vi "Trigger Each Line From Encoder (Camera Link).vi"() -> ()   [LabVIEW 2023]
doc: "The Trigger Each Line From Encoder (Camera Link) VI uses the Phase A & B pins from an encoder to trigger the acquisition of each image line. Because the encoder frequency is generally higher than the desired line rate, use the Divide Factor to adjust the Scaled Encoder signal frequency to match that of the desired line rate. The encoder hardware on NI frame grabbers is designed to accomodate backlash, so the Scaled Encoder signal will only pulse for cumulative forward movement of the encoder itself.\n\nNOTE: This example requires a linescan camera with an IMAQdx-supported Camera Link frame grabber. If supported, the Use IO Board Input control determines whether the encoder input lines are sourced from the IO Extension Board or from the front panel IO connector."
uses:
  <vilib>/vision/driver/NI_Vision_Acquisition_Software.lvlib
  <resource>/objmgr/imaqdx.rc
panel:
  in  "Encoder Parameters":T1={"Divide Factor"=10, "Phase A Polarity"=0, "Phase B Polarity"=0, "Phase A & B Filter"=FALSE, "Use IO Board Input"=FALSE} {"Phase B Polarity" items=["Active High", "Active Low"]; "Phase A Polarity" items=["Active High", "Active Low"]}
  in  "Camera Name":refnum<k21> caption="IMAQdx Session"
  out "Buffer Number":u32
  out "Image":T2(plugin-control)
  out "Frame Rate":dbl
  in  "Stop":bool
  # "Overview: Demonstrates how to acquire images continuously using a grab acquisition while triggering each line of an image from an encoder.\nRequirements: Vision Acquisition Software; Camera Link frame grabber; Camera Link line scan camera configured to trigger each line from Camera Control line 1 (CC1); encoder wired to the encoder input of the frame grabber\nInstructions: \n1. Select the Camera Name.\n2. Configure the encoder parameters.\n3. Run the VI"
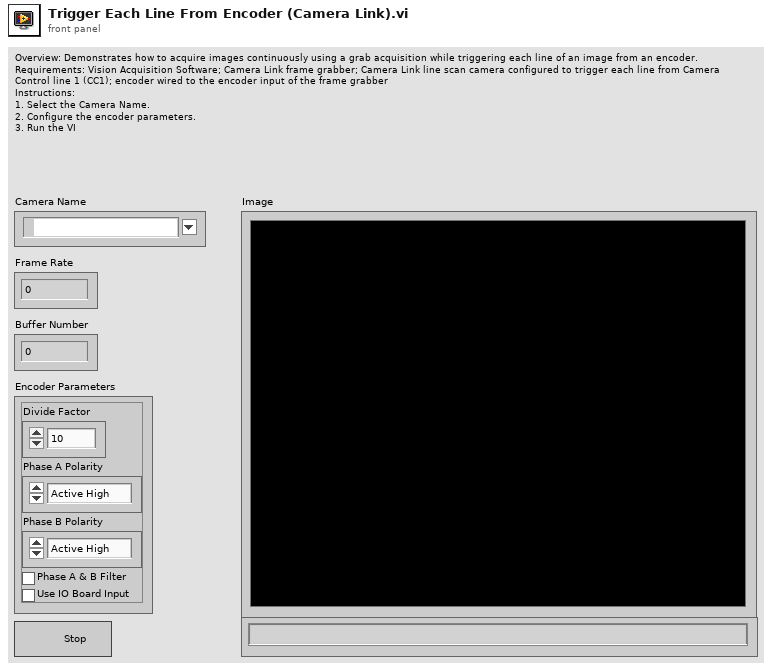
[diagram p1: front panel]
types:
  T1 = cluster{"Divide Factor":u32, "Phase A Polarity":u32, "Phase B Polarity":u32, "Phase A & B Filter":bool, "Use IO Board Input":bool}
  T2 = typedef "IMAQ Image.ctl" = refnum<image>
  T3 = typedef "IMAQdx.ctl" = refnum<k21>
  T4 = enum8{"Enabled", "Disabled", "Disabled and Grayed Out"}
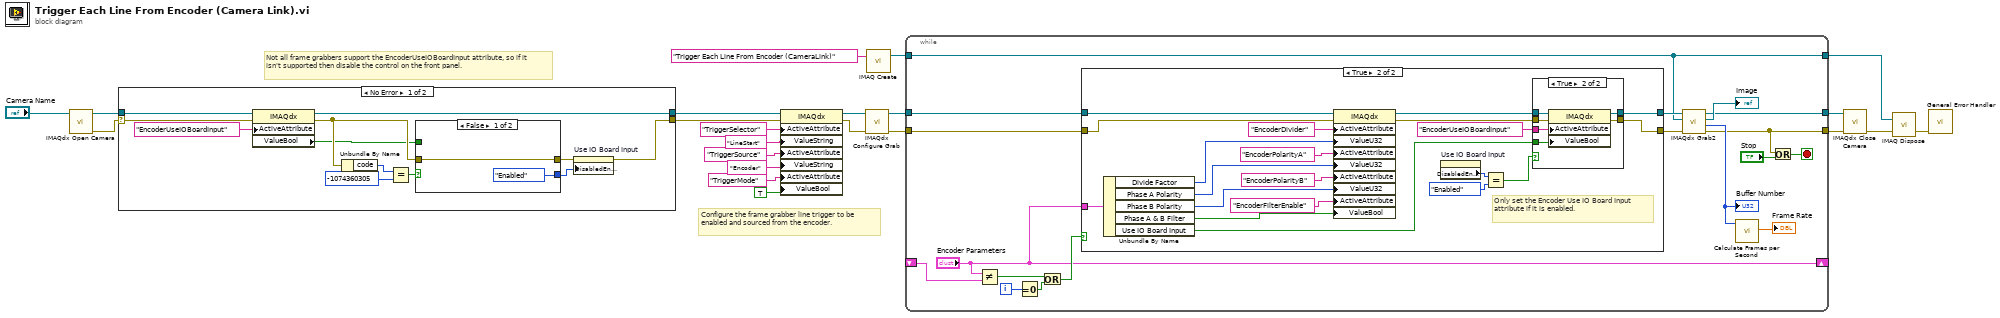
[diagram p0: block diagram]
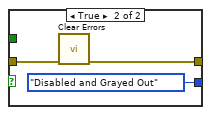
[diagram p4: hidden frame]
diagram:
  # "Configure the frame grabber line trigger to be enabled and sourced from the encoder."
  # "Not all frame grabbers support the EncoderUseIOBoardInput attribute, so if it isn't supported then disable the control on the front panel."
  n1 = call <vilib>:"IMAQdx Open Camera.vi"("Session In"="Camera Name") -> ("error out"=w5:errorcluster, "Session Out"=w6:T3)  [unwired: 2 in, 7 out]
  n2 = case shown="No Error" w5 {
    selector: w5 -> [w31 w40]
    tunnel: w6 -> [w33 w41]
    tunnel: [w32 w41] -> w2
    tunnel: [w25 w40] -> w1
    frame No Error {
      n3 = property class="IMAQdx"(reference=w33, error in=w31, "ActiveAttribute"="EncoderUseIOBoardInput") -> (reference out=w32:T3, error out=w28:errorcluster, "ValueBool"=w23:bool)
      n4 = Unbundle By Name(w28) -> ("code"=w30:i32)
      n5 = Equal?(x=w30, y=-1074360305) -> (x = y?=w24:bool)
      n6 = case shown="False" w24 {
        tunnel: w28 -> [w36 w39]
        tunnel: [w36 w38] -> w27
        tunnel: [T4."Enabled" ("Disabled") T4."Disabled and Grayed Out" ("Disabled")] -> w26
        tunnel: w23 -> [_ _]
        frame False {
        }
        frame True {
          n7 = call <vilib>:"Clear Errors.vi"("error in (no error)"=w39) -> ("error out"=w38:errorcluster)  [unwired: 5 in, 1 out]
        }
      }
      n8 = property on="Use IO Board Input" class="Bool (strict)"(error in=w27, "DisabledEnum"=w26) -> (error out=w25:errorcluster)  [unwired: 1 in, 1 out]
    }
    frame Error {
    }
  }
  n9 = property class="IMAQdx"(reference=w2, error in=w1, "ActiveAttribute"="TriggerSelector", "ValueString"="LineStart", "ActiveAttribute"="TriggerSource", "ValueString"="Encoder", "ActiveAttribute"="TriggerMode", "ValueBool"=TRUE) -> (reference out=w4:T3, error out=w3:errorcluster)
  n10 = call <vilib>:"IMAQdx Configure Grab.vi"("error in"=w3, "Session In"=w4) -> ("error out"=w7:errorcluster, "Session Out"=w8:T3)  [unwired: 8 in]
  n11 = call "IMAQ Create"("Image Name"="Trigger Each Line From Encoder (CameraLink)") -> ("New Image"=w22:T2)  [unwired: 3 in, 2 out]
  n12 = while {
    tunnel: [w44] -> w21
    tunnel: [w55] -> w20
    tunnel: w22 -> [w42]
    tunnel: [w42] -> w18
    shift-right: ["Encoder Parameters"] -> _
    shift-left: _ -> [w49]
    tunnel: w8 -> [w46]
    tunnel: w7 -> [w45]
    i -> [w52]
    stop <- w59 stop-if-true
    n13 = Not Equal?(x="Encoder Parameters", y=w49) -> (x != y?=w53:bool)
    n14 = Equal To 0?(x=w52) -> (x = 0?=w51:bool)
    n15 = Or(x=w53, y=w51) -> (x .or. y?=w50:bool)
    n16 = case shown="True" w50 {
      tunnel: "Encoder Parameters" -> [_ w81]
      tunnel: [w61 w63] -> w48
      tunnel: [w60 w62] -> w47
      tunnel: w46 -> [w61 w72]
      tunnel: w45 -> [w60 w71]
      frame False {
      }
      frame True {
        # "Only set the Encoder Use IO Board Input attribute if it is enabled."
        n17 = Unbundle By Name(w81) -> ("Divide Factor"=w79:u32, "Phase A Polarity"=w77:u32, "Phase B Polarity"=w75:u32, "Phase A & B Filter"=w73:bool, "Use IO Board Input"=w65:bool)
        n18 = property class="IMAQdx"(reference=w72, error in=w71, "ActiveAttribute"="EncoderDivider", "ValueU32"=w79, "ActiveAttribute"="EncoderPolarityA", "ValueU32"=w77, "ActiveAttribute"="EncoderPolarityB", "ValueU32"=w75, "ActiveAttribute"="EncoderFilterEnable", "ValueBool"=w73) -> (reference out=w70:T3, error out=w69:errorcluster)
        n19 = property on="Use IO Board Input" class="Bool (strict)"() -> ("DisabledEnum"=w68:T4)  [unwired: 2 in, 2 out]
        n20 = Equal?(x=w68, y=T4."Enabled" ("Disabled")) -> (x = y?=w64:bool)
        n21 = case shown="True" w64 {
          tunnel: w70 -> [w82 w89]
          tunnel: w69 -> [w83 w88]
          tunnel: "EncoderUseIOBoardInput" ("ActiveAttribute") -> [_ w87]
          tunnel: w65 -> [_ w86]
          tunnel: [w82 w85] -> w63
          tunnel: [w83 w84] -> w62
          frame False {
          }
          frame True {
            n22 = property class="IMAQdx"(reference=w89, error in=w88, "ActiveAttribute"=w87, "ValueBool"=w86) -> (reference out=w85:T3, error out=w84:errorcluster)
          }
        }
      }
    }
    n23 = call <vilib>:"IMAQdx Grab2.vi"("error in"=w47, "Image In"=w42, "Session In"=w48) -> ("error out"=w55:errorcluster, "Buffer Number Out"=w56:u32, "Image Out"=→"Image":T2, "Session Out"=w44:T3)  [unwired: 5 in]
    "Buffer Number" <- w56
    n24 = call <vilib>:"Calculate Frames per Second.vi"("Buffer Number"=w56) -> ("Processed Frames/s"=→"Frame Rate":dbl)  [unwired: 8 in, 2 out]
    n25 = Or(x=w55, y="Stop") -> (x .or. y?=w59:bool)
  }
  n26 = call <vilib>:"IMAQdx Close Camera.vi"("error in"=w20, "Session In"=w21) -> ("error out"=w17:errorcluster)  [unwired: 9 out]
  n27 = call "IMAQ Dispose"("Image"=w18, "error in (no error)"=w17) -> ("error out"=w16:errorcluster)  [unwired: 4 in]
  n28 = call <vilib>:"General Error Handler.vi"("error in (no error)"=w16) -> ()  [unwired: 2 in, 13 out]
